vi "Vision Test.vi"() -> ()   [LabVIEW 2011]
panel:
  out "Shape Report (Shape Matching 1)":T1(array[cluster]) {"Score" format="%.2f"; "Centroid"."y" format="%.2f"; "Centroid"."x" format="%.2f"}
  out "Number of Matches (Shape Matching 1)":i32
  out "Image Number":u32
  out "Frame Rate":dbl
  in  "Stop (F)":bool
  out "Image Out 2":T2(plugin-control)
  out "Image Out":T2(plugin-control)
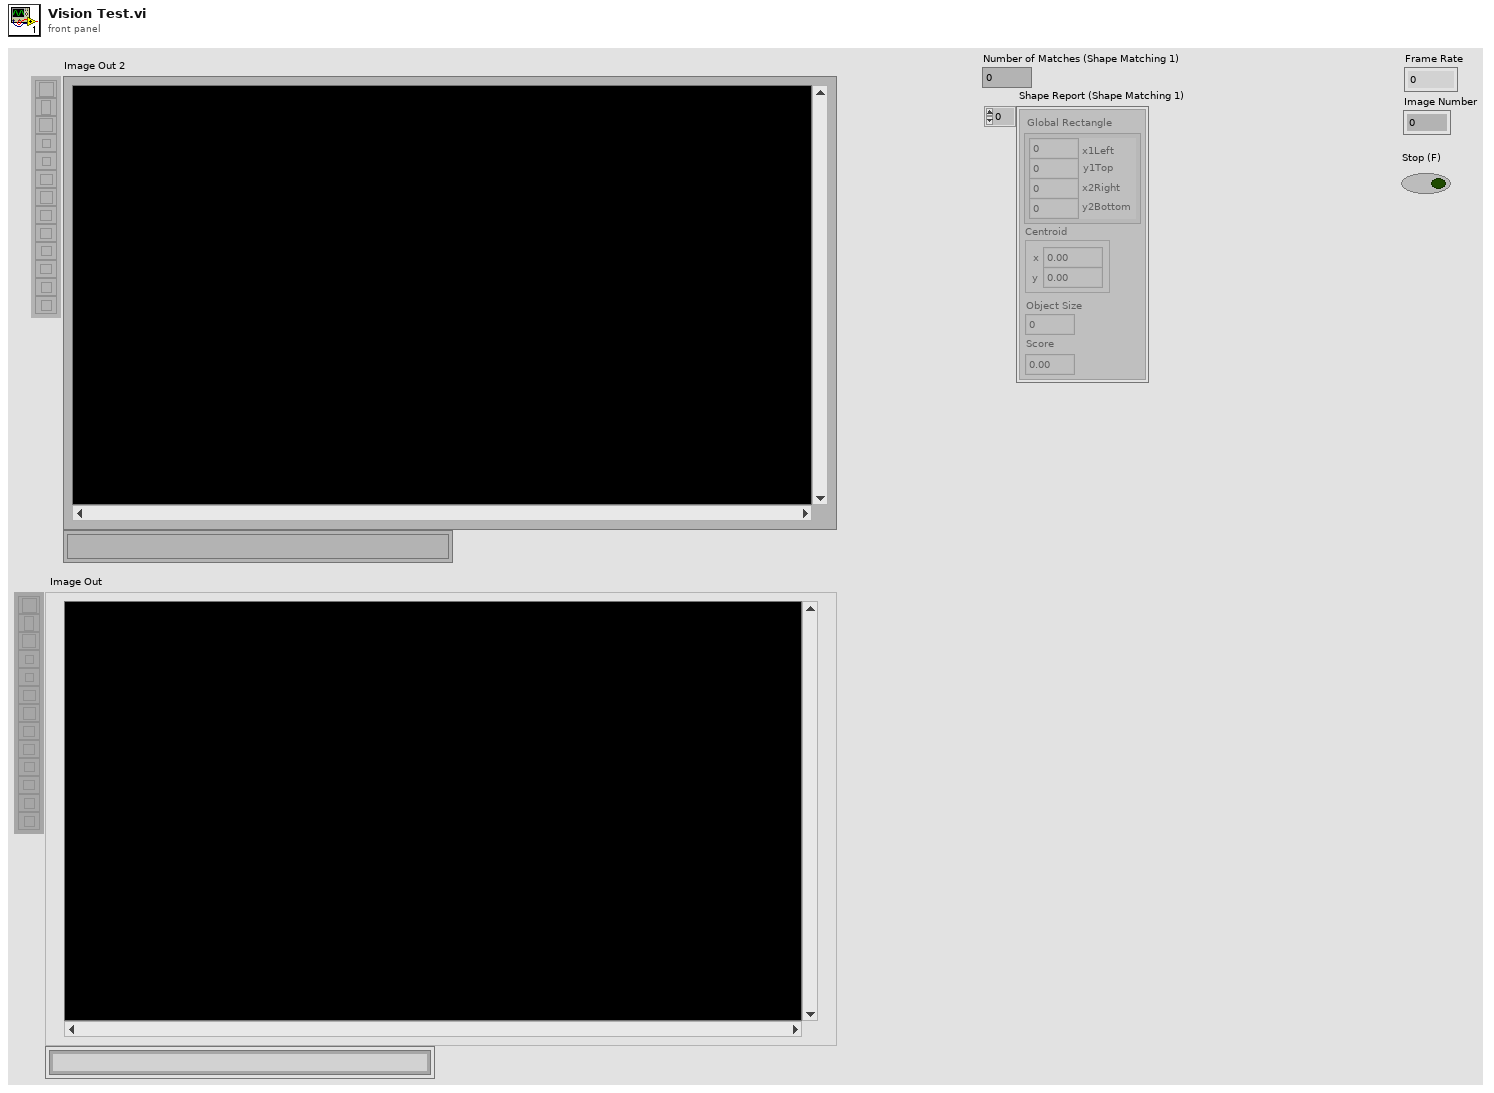
[diagram p1: front panel]
types:
  T1 = cluster{"Global Rectangle":cluster{"x1Left":i32, "y1Top":i32, "x2Right":i32, "y2Bottom":i32}, "Centroid":cluster{"x":sgl, "y":sgl}, "Object Size":u32, "Score":dbl}[]
  T2 = typedef "IMAQ Image.ctl" = refnum<image>
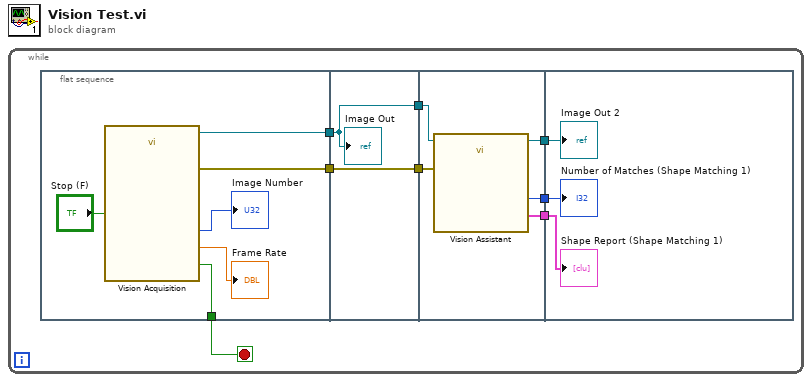
[diagram p0: block diagram]
diagram:
  n1 = while {
    stop <- w8 stop-if-true
    n2 = flat-sequence {
      tunnel: [w13] -> w8
      tunnel: [w10] -> w7
      tunnel: [w9] -> w5
      tunnel: w7 -> [w16]
      tunnel: [w16] -> w6
      tunnel: w5 -> [w15]
      tunnel: [w15] -> w4
      tunnel: w6 -> [w21]
      tunnel: w4 -> [w20]
      tunnel: [w19] -> w3
      tunnel: [w18] -> w2
      tunnel: [w17] -> w1
      tunnel: w3 -> [w24]
      tunnel: w2 -> [w23]
      tunnel: w1 -> [w22]
      frame #0 {
        n3 = call "Vision Acquisition"("Stop (F)"="Stop (F)") -> ("Image Out"=w10:T2, "Image Number"=→"Image Number":u32, "Frame Rate"=→"Frame Rate":dbl, "Stopped"=w13:bool, "error out"=w9:errorcluster)  [unwired: 22 in]
      }
      frame #1 {
        "Image Out" <- w16
      }
      frame #2 {
        n4 = call "Vision Assistant"("Image In"=w21, "error in"=w20) -> ("Image Out"=w19:T2, "Number of Matches (Shape Matching 1)"=w18:i32, "Shape Report (Shape Matching 1)"=w17:T1)  [unwired: 22 in, 1 out]
      }
      frame #3 {
        "Image Out 2" <- w24
        "Number of Matches (Shape Matching 1)" <- w23
        "Shape Report (Shape Matching 1)" <- w22
      }
    }
  }
